vi "Get Direct Sampling State.vi"(8 "error in (no error)":errorcluster, 11 "DeviceRefnum":u64) -> (0 "error out":errorcluster, 2 "Direct Sampling State":T1, 3 "DeviceRefnum Out":u64)   [LabVIEW 2016]
doc: "Gets the state if the direct sampling mode."
uses:
  Controls/Direct Sampling States.ctl
panel:
  out "function return":i32
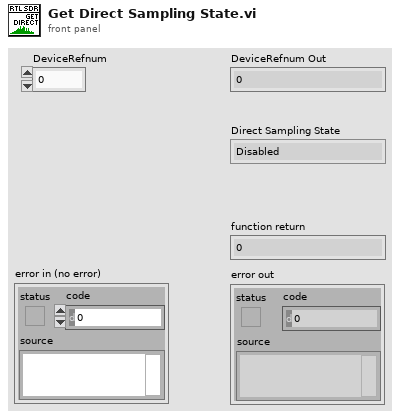
[diagram p1: front panel]
types:
  T1 = typedef "Direct Sampling States.ctl" = enum16{"Disabled", "I-ADC Input Enabled", "Q-ADC Input Enabled"}
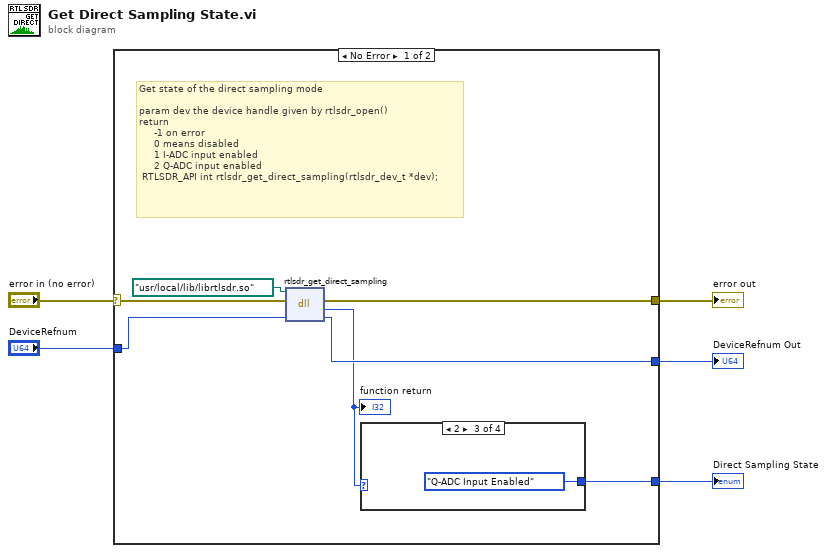
[diagram p0: block diagram]
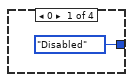
[diagram p2: hidden frame]
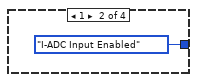
[diagram p3: hidden frame]
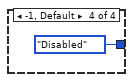
[diagram p4: hidden frame]
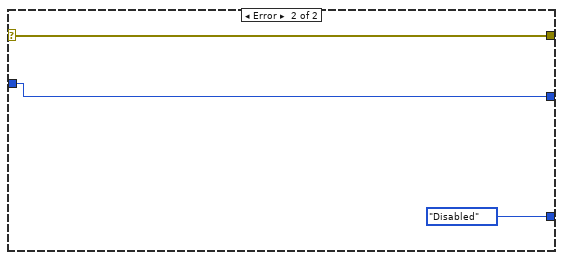
[diagram p5: hidden frame]
diagram:
  n1 = case shown="No Error" "error in (no error)" {
    selector: "error in (no error)" -> [w7 w17]
    tunnel: "DeviceRefnum" -> [w11 w19]
    tunnel: [w10 w19] -> w4
    tunnel: [w8 Direct_Sampling_States."Disabled"] -> w3
    tunnel: [w6 w17] -> w1
    frame No Error {
      # "Get state of the direct sampling mode\n\nparam dev the device handle given by rtlsdr_open()\nreturn \n     -1 on error\n     0 means disabled  \n     1 I-ADC input enabled\n     2 Q-ADC input enabled\n RTLSDR_API int rtlsdr_get_direct_sampling(rtlsdr_dev_t *dev);"
      n2 = dll-call lib="C:/Program Files (x86)/National Instruments/LabVIEW 2016/user.lib/rtlsdr/rtlsdr.*" fn="rtlsdr_get_direct_sampling"(path in=path "/usr/local/lib/librtlsdr.so", error in=w7, "DeviceRefnum"=w11) -> (error out=w6:errorcluster, "return type"=w9:i32, "DeviceRefnum"=w10:u64)  [unwired: 1 in, 1 out]
      "function return" <- w9
      n3 = case shown="2" w9 {
        tunnel: [Direct_Sampling_States."Disabled" Direct_Sampling_States."I-ADC Input Enabled" Direct_Sampling_States."Q-ADC Input Enabled" Direct_Sampling_States."Disabled"] -> w8
        frame 0 {
        }
        frame 1 {
        }
        frame 2 {
        }
        frame -1, Default {
        }
      }
    }
    frame Error {
    }
  }
  "DeviceRefnum Out" <- w4
  "Direct Sampling State" <- w3
  "error out" <- w1
